vi "get file info.vi"(8 "error in":errorcluster, 11 "Picture File in":refnum<class "Picture File.lvclass">) -> (0 "error out":errorcluster, 3 "Picture File out":refnum<class "Picture File.lvclass">)   [LabVIEW 2023, in "File Classes.lvlib" / "Picture File.lvclass"]
uses:
  Picture File.lvclass
  D:/Library/LabVIEW Projects/Personal projects/Picture Organiser/PictureOrganizer/File Classes/File/File.lvclass
  File/File.lvclass/File.ctl
  Picture File.lvclass/Picture File.ctl
  File/Accessors/Read Source Path.vi
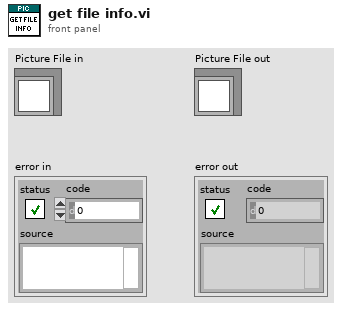
[diagram p1: front panel]
types:
  T1 = typedef "File Classes.lvlib/exif data cluster.ctl" = cluster{"Make":string, "Model":string, "Orientation":u16, "Date":timestamp, "Width":u16, "Height":u16, "Square?":bool, "File Name":string, "Extension":string, "Valid?":bool, "Path":path, "size":i64, "No Ext?":bool, "prefix?":bool, "Tag":string, "Name Type":T2, "Projection Type":string}
  T2 = typedef "File Classes.lvlib/rename type enum.ctl" = enum16{"Date & Time (Default)", "Model Sufix", "Event Sufix", "Model & Event Sufix"}
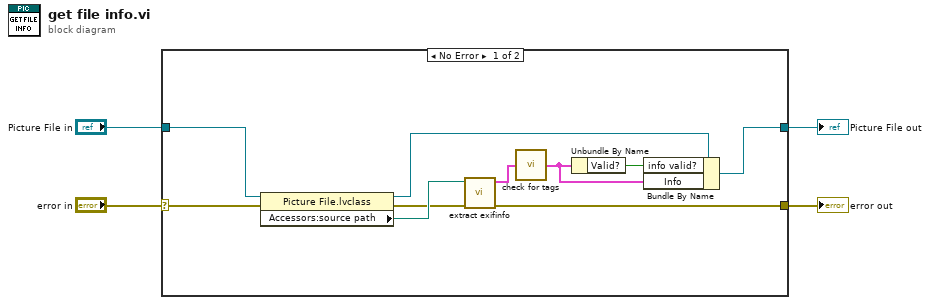
[diagram p0: block diagram]
diagram:
  n1 = case shown="No Error" "error in" {
    selector: "error in" -> [w13 w15]
    tunnel: "Picture File in" -> [w14 w16]
    tunnel: [w8 w16] -> w2
    tunnel: [w10 w15] -> w1
    frame No Error {
      n2 = property class="Picture File.lvclass"(reference=w14, error in=w13) -> (reference out=w9:refnum<class "Picture File.lvclass">, error out=w11:errorcluster, "Accessors:source path"=w12:path)
      n3 = call "extract exifinfo.vi"("error in"=w11, "file path"=w12) -> ("error IO"=w10:errorcluster, "Info"=w6:T1)  [unwired: 8 in]
      n4 = call "check for tags.vi"("Info"=w6) -> ("Info 2"=w5:T1)
      n5 = Unbundle By Name(w5) -> ("Valid?"=w7:bool)
      n6 = Bundle By Name(cluster=w9, "info valid?"=w7, "Info"=w5) -> (w8:refnum<class "Picture File.lvclass">)
    }
    frame Error {
    }
  }
  "error out" <- w1
  "Picture File out" <- w2
